vi "Test Create (From Structure).vi"(8 "error in (no error)":errorcluster) -> (0 "error out":errorcluster)   [LabVIEW 2020, in "TEST JKI State Machine API.lvlib"]
uses:
  TEST JKI State Machine API.lvlib
  source/JKI SM/JKI SM.lvclass
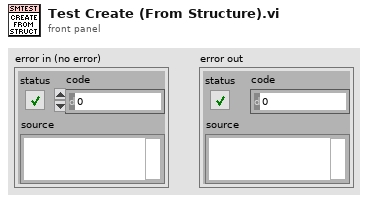
[diagram p1: front panel]
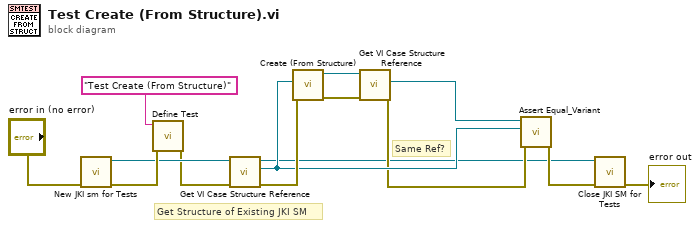
[diagram p0: block diagram]
diagram:
  # "Same Ref?"
  # "Get Structure of Existing JKI SM"
  n1 = call "New JKI sm for Tests.vi"("error in (no error)"="error in (no error)") -> ("error out"=w14:errorcluster, "JKI SM out"=w9:refnum<class "JKI SM.lvclass">)  [unwired: 9 in]
  n2 = call <vilib>:"Define Test.vi"("error in (no error)"=w14, "Label (VI Title)"="Test Create (From Structure)") -> ("error out"=w8:errorcluster)  [unwired: 8 in, 1 out]
  n3 = call "Get VI Case Structure Reference.vi"("error in (no error)"=w8, "JKI SM in"=w9) -> ("error out"=w5:errorcluster, "Case Structure ref"=w3:refnum<vi>, "JKI SM out"=w1:refnum<class "JKI SM.lvclass">)  [unwired: 7 in]
  n4 = call "Create (From Structure).vi"("error in (no error)"=w5, "Structure"=w3) -> ("error out"=w6:errorcluster, "JKI SM out"=w7:refnum<class "JKI SM.lvclass">)  [unwired: 8 in]
  n5 = call "Get VI Case Structure Reference.vi"("error in (no error)"=w6, "JKI SM in"=w7) -> ("error out"=w2:errorcluster, "Case Structure ref"=w4:refnum<vi>)  [unwired: 7 in, 1 out]
  n6 = call <vilib>:"Assert Equal_Variant.vi"("error in (no error)"=w2, "Y"=w3, "X"=w4) -> ("error out"=w11:errorcluster)  [unwired: 8 in]
  n7 = call "Close JKI SM for Tests.vi"("error in (no error)"=w11, "JKI SM in"=w1) -> ("error out"=→"error out":errorcluster)  [unwired: 9 in]
